vi "New Log File.vi"(7 "Log File Type":refnum<class "Log File.lvclass">, 8 "error in (no error)":errorcluster, 9 "Disable Buffering (F)":bool, 10 "Operation":T1, 11 "File Path":path) -> (0 "error out":errorcluster, 3 "Log File out":refnum<class "Log File.lvclass">)   [LabVIEW 2015, in "Waveform Data Logger Engine.lvlib" / "Log File.lvclass"]
uses:
  Log File.lvclass
  Operation.ctl
  Log File.lvclass/Log File.ctl
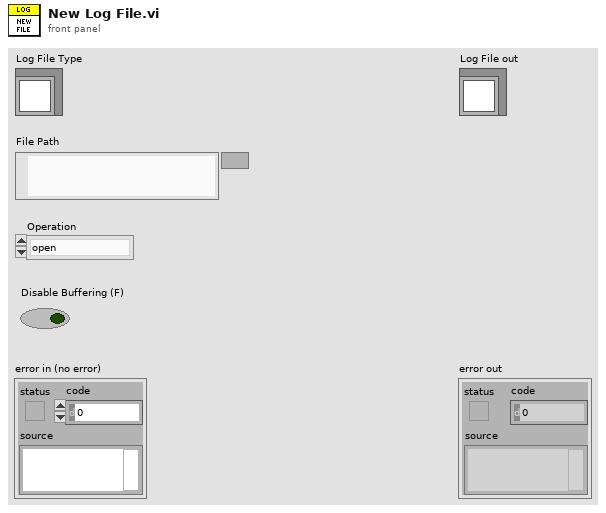
[diagram p1: front panel]
types:
  T1 = typedef "Waveform Data Logger Engine.lvlib/Log File.lvclass/Operation.ctl" = enum16{"open", "open or create", "create or replace", "create", "open (read-only)"}
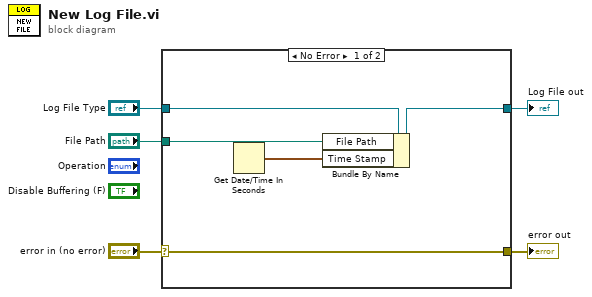
[diagram p0: block diagram]
diagram:
  n1 = case shown="No Error" "error in (no error)" {
    selector: "error in (no error)" -> [w9 w12]
    tunnel: [w9 w12] -> w4
    tunnel: [w8 w11] -> w2
    tunnel: "Log File Type" -> [w10 w11]
    tunnel: "File Path" -> [w7 _]
    frame No Error {
      n2 = Get Date/Time In Seconds() -> (seconds since 1Jan1904=w6:timestamp)
      n3 = Bundle By Name(cluster=w10, "File Path"=w7, "Time Stamp"=w6) -> (w8:refnum<class "Log File.lvclass">)
    }
    frame Error {
    }
  }
  "error out" <- w4
  "Log File out" <- w2
